vi "Target_425.vi"() -> ()   [LabVIEW 2018]
uses:
  <vilib>/Platform/TimedLoop/XDataNode/timing_clust.ctl
  <vilib>/Platform/TimedLoop/XDataNode/nitl_modes.ctl
  <vilib>/Platform/TimedLoop/XDataNode/wakeup.ctl
  <vilib>/rvi/eio/common/nirviEmuTemplateMethod_errors.vi
  <vilib>/rvi/Emulation/niFpgaSctlEmulationGetInTimedLoop.vi
  <vilib>/rvi/Emulation/niFpgaEmulationReportErrorSimple.vi
  <vilib>/rvi/Emulation/niFpgaGetClockAttributes.vi
  <vilib>/rvi/Emulation/niFpgaCriticalErrorInLSC.vi
  <vilib>/rvi/Emulation/niFpgaProcessEmulError.vi
  <vilib>/rvi/interface/RandomDataEmulation/niFpgaRandomDataHandleErrors.vi
  <vilib>/rvi/Memory/Memory_Emulation/nirvimemoryEmulation.vi
  <vilib>/rvi/Memory/Memory_Emulation/nirvimemoryFastEmulation.vi
  <vilib>/rvi/DataTransferAndStorage/Container/Common/niFpgaContainerGetUniqueNameForEmu.vi
  <vilib>/rvi/Memory/Memory_Emulation/niFpgaMemoryEmulationCacheClearOnFirstRun.vi
  <vilib>/rvi/Memory/Memory_Emulation/nirvimemoryEmulationManagerCache_MakeExclusive.vi
  <vilib>/rvi/Memory/Memory_Emulation/niFpgaMemoryEmulationValidateCache.vi
  <vilib>/rvi/Memory/Memory_Emulation/nirvimemoryEmulationManagerCache_InsertValue.vi
  <vilib>/Utility/error.llb/Clear Errors.vi
  <vilib>/rvi/Memory/Memory_Emulation/nirvimemoryEmulationManagerCache_ReleaseExclusive.vi
  <vilib>/rvi/Memory/Memory_Emulation/nirvimemoryEmulationManagerCache_GetValue.vi
  <vilib>/rvi/Emulation/niFpgaEmulationIsFPGAContextNoSignature.vi
  <vilib>/rvi/Memory/Memory_Emulation/nirvimemoryEmulationManagerCache_SetValue.vi
  <vilib>/rvi/Emulation/niFpgaSctlEmulationResourceMgr.vi
  <vilib>/eio/EIONode/EIONode.xnode
  <vilib>/Platform/TimedLoop/XDataNode/XDataNode.xnode
  <vilib>/rvi/DataTransferAndStorage/Container/XNode/niFpgaContainer.xnode
  <vilib>/rvi/interface/RandomDataEmulation/nirviRandomDataFpgaReadWriteTemplate.vi
  <vilib>/Platform/TimedLoop/XDataNode/XDNodeRunTimeDep.lvlib
  <vilib>/rvi/Memory/Memory_Emulation/niFpgaMemoryFastEmulationDramWriteAndRequestData.vi
  <vilib>/rvi/Memory/Memory_Emulation/niFpgaMemoryEmulationDramWriteAndRequestData.vi
  <instrlib>/_niInstr/Basic Elements/v1/FPGA/niInstr Basic Elements v1 FPGA.lvlib
  <vilib>/rvi/Memory/Memory_Emulation/niFpgaMemoryEmulationDramRetrieveData.vi
panel:
  in  "30":u8=30
  in  "4":u8=4
  in  "20":u8=20
  in  "3":u8=3
  in  "28":u8=28
  in  "2":u8=2
  out "XVS":bool
  out "XHS":bool
  out "TOUT0":bool
  out "TOUT1":bool
  out "TOUT2":bool
  in  "OMODE":bool
  in  "XTRIG2":bool
  in  "XTRIG1":bool
  in  "XMASTER":bool
  in  "Хватит":bool
  in  "48":bool[](array[boolean])=[FALSE, FALSE, FALSE, FALSE, FALSE, FALSE, FALSE, FALSE, FALSE, FALSE, FALSE, FALSE, FALSE, FALSE, FALSE, FALSE, FALSE, FALSE, FALSE, FALSE, FALSE, FALSE, FALSE, FALSE, FALSE, FALSE, FALSE, FALSE, FALSE, FALSE, FALSE, FALSE, FALSE, FALSE, FALSE, FALSE, FALSE, FALSE, FALSE, FALSE, FALSE, FALSE, FALSE, FALSE, FALSE, FALSE, FALSE, FALSE]
  in  "48":u8=48
  out "Записали адресов":u32
  in  "3445760":u32=3445760
  in  "Стоп":bool
  in  "4-wire":bool
  in  "W(T)/R(F)":bool
  in  "Адрес":u8
  in  "Кол-во":u16=185
  in  "185":u16=185
  in  "187":u16=187
  in  "184":u16=184
  in  "Upd_RD":bool
  in  "Upd_WR":bool
  in  "XCLR":bool
  in  "Автомат":bool
  in  "Кадр в память":bool
  in  "Кадр на ПК":bool
  in  "Нач_адр":u32
  in  "Кон_адр":u32=26920
  out "Записали FIFO":bool
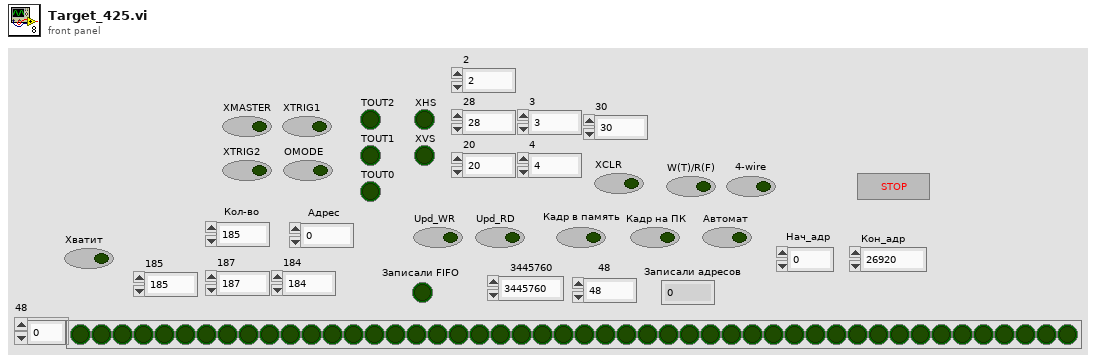
[diagram p1: front panel]
types:
  T1 = typedef "XDNodeRunTimeDep.lvlib/timing_clust.ctl" = cluster{"Expected End [f-1]":u64, "Actual End [f-1]":u64, "Finished Late? [f-1]":bool, "Expected End [i-1]":u64, "Actual End [i-1]":u64, "Finished Late? [i-1]":bool, "Expected Start [i]":u64, "Actual Start [i]":u64, "Expected Start [f]":u64, "Actual Start [f]":u64, "Source Name":string, "Structure Name":string, "Period":i64, "Deadline":i64, "Offset":i64, "Start":i64, "Priority":i32, "Timeout":i32, "Mode":T2, "Wakeup Reason":T3, "Error":errorcluster, "Source Type":string, "Secondary Source Type":string, "Global End Time":u64, "Global Start Time":u64, "Frame Duration":u64, "Iteration Duration":u64, "Assigned CPU":i32, "I/O Scan Engine Mode":u32}
  T2 = typedef "XDNodeRunTimeDep.lvlib/nitl_modes.ctl" = enum32{"No Change", "Process missed periods, maintain original phase", "Discard missed periods, maintain original phase", "Process missed periods, ignore original phase", "Discard missed periods, ignore original phase"}
  T3 = typedef "XDNodeRunTimeDep.lvlib/wakeup.ctl" = enum32{"Normal", "Aborted", "Asynchronous wakeup", "Timing source error", "Timed loop error", "Timeout"}
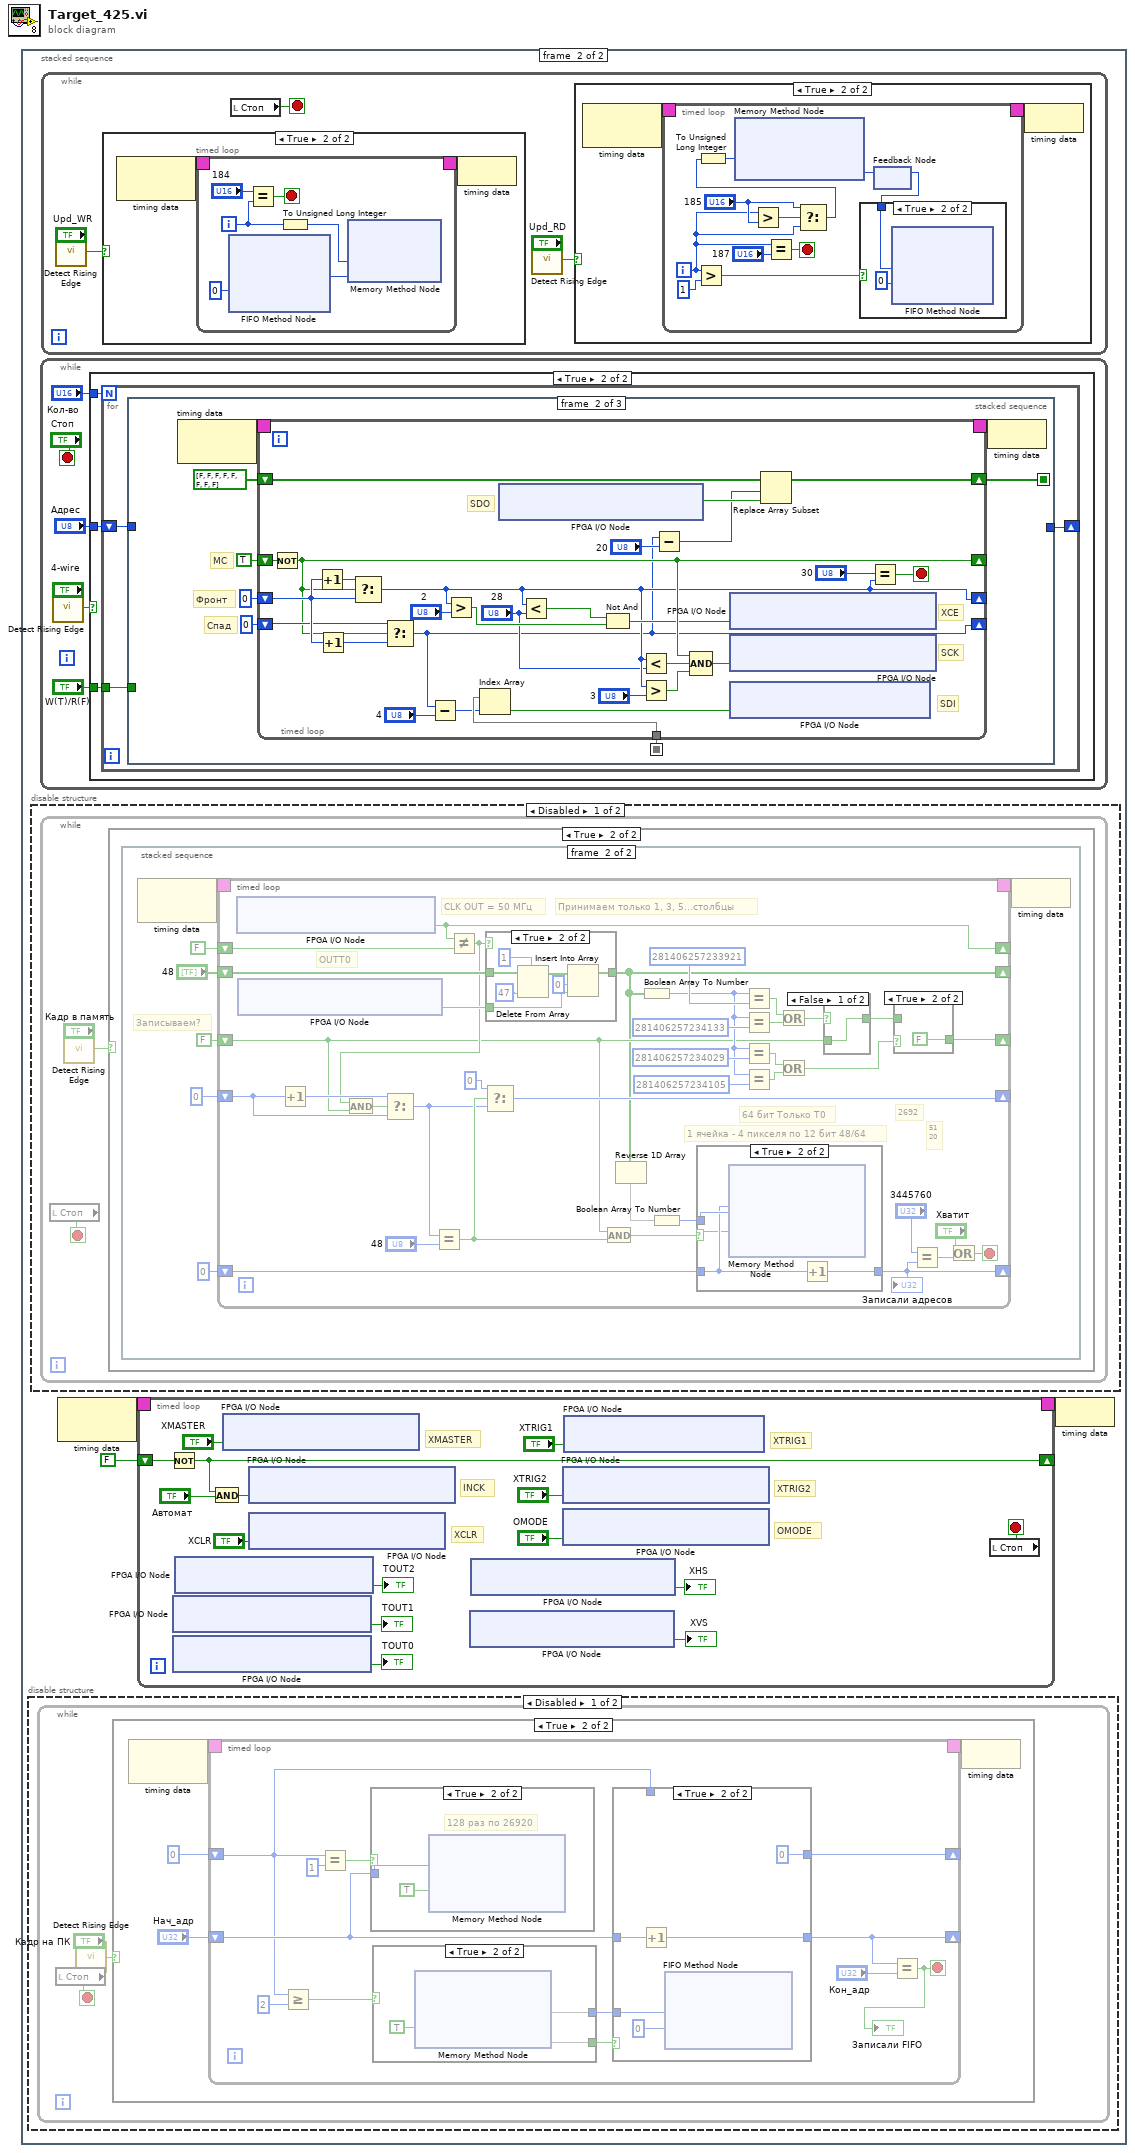
[diagram p0: block diagram]
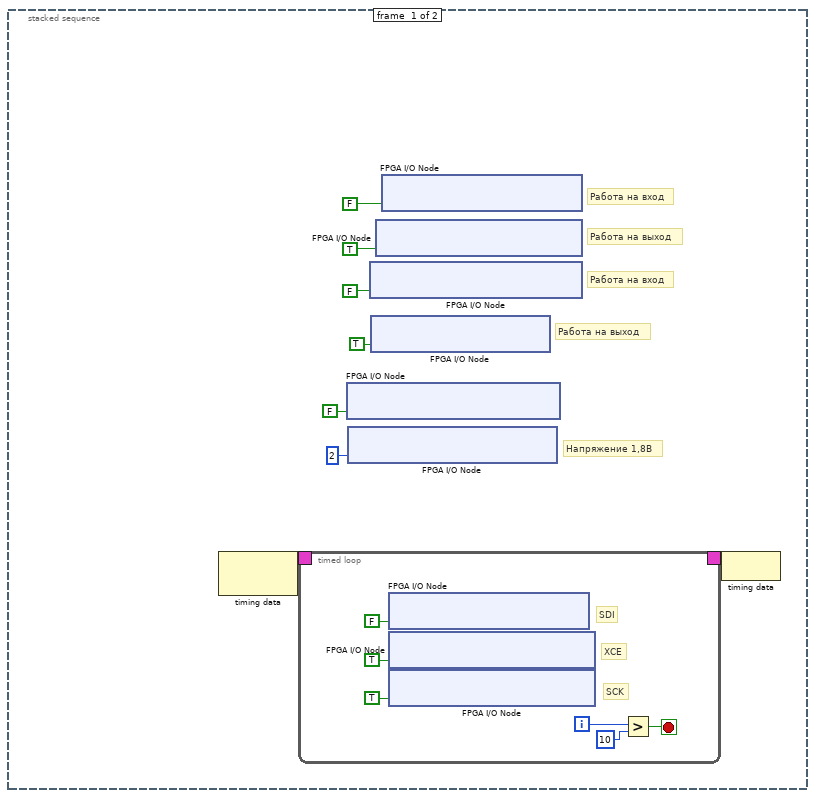
[diagram p2: hidden frame]
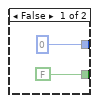
[diagram p4: hidden frame]
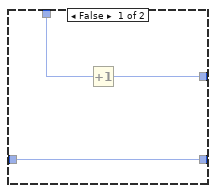
[diagram p6: hidden frame]
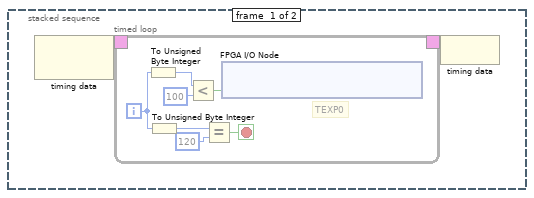
[diagram p9: hidden frame]
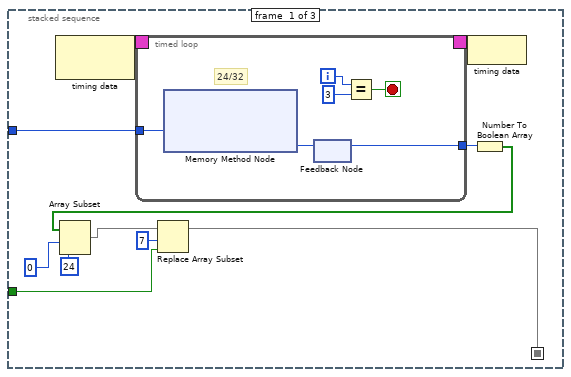
[diagram p16: hidden frame]
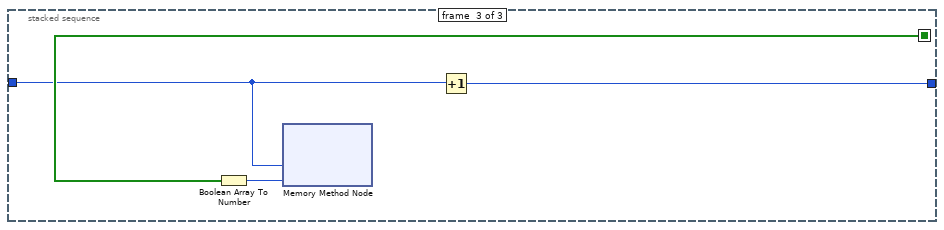
[diagram p17: hidden frame]
diagram:
  n1 = stacked-sequence {
    frame #0 {
      # "Напряжение 1,8В"
      # "Работа на выход"
      # "Работа на вход"
      # "Работа на выход"
      # "Работа на вход"
      n2 = node-c288() -> (w2:T1)  [unwired: 1 in]
      n3 = timed-loop {
        timing: w2 -> [_]
        timing-out: [_] -> w1
        i -> [w11]
        stop <- w9 stop-if-true
        # "SCK"
        # "XCE"
        # "SDI"
        n4 = xnode "FPGA I/O Node"("IO Module\\DDCA_DIO9_Write"=FALSE ("IO Module\\DDCA_DIO9_Write")) -> ()  [unwired: 1 in, 1 out]
        n5 = xnode "FPGA I/O Node"("IO Module\\DDCA_DIO13_Write"=TRUE ("IO Module\\DDCA_DIO13_Write")) -> ()  [unwired: 1 in, 1 out]
        n6 = xnode "FPGA I/O Node"("IO Module\\DDCA_DIO15_Write"=TRUE ("IO Module\\DDCA_DIO15_Write")) -> ()  [unwired: 1 in, 1 out]
        n7 = Greater?(x=w11, y=u8 10) -> (0:w9:bool)
      }
      n8 = xnode "FPGA I/O Node"("IO Module\\DDCA_Supply_Select"=FALSE ("IO Module\\DDCA_Supply_Select")) -> ()  [unwired: 1 in, 1 out]
      n9 = xnode "FPGA I/O Node"("IO Module\\Local_Supply_Select"=u8 2 ("IO Module\\Local_Supply_Select")) -> ()  [unwired: 1 in, 1 out]
      n10 = xnode "FPGA I/O Node"("IO Module\\DDCA_DIO16-23_WE"=FALSE ("IO Module\\DDCA_DIO16-23_WE")) -> ()  [unwired: 1 in, 1 out]
      n11 = xnode "FPGA I/O Node"("IO Module\\DDCA_PFI_WE"=TRUE ("IO Module\\DDCA_DIO16-23_WE")) -> ()  [unwired: 1 in, 1 out]
      n12 = xnode "FPGA I/O Node"("IO Module\\DDCA_DIO8-15_WE"=TRUE ("IO Module\\DDCA_DIO8-15_WE")) -> ()  [unwired: 1 in, 1 out]
      n13 = xnode "FPGA I/O Node"("IO Module\\DDCA_DIO0-7_WE"=FALSE ("IO Module\\DDCA_DIO0-7_WE")) -> ()  [unwired: 1 in, 1 out]
      n14 = node-c288(w1) -> ()
    }
    frame #1 {
      n15 = disable-structure shown="Disabled" {
        frame Disabled {
          n16 = while {
            stop <- w24 stop-if-true
            n17 = local read "Стоп"() -> (w24:bool)
            n18 = call <instrlib>:"Detect Rising Edge.vi"("signal"="Кадр на ПК") -> ("edge detected"=w23:bool)  [unwired: 14 in]
            n19 = case shown="True" w23 {
              frame False {
              }
              frame True {
                n20 = node-c288() -> (w28:T1)  [unwired: 1 in]
                n21 = timed-loop {
                  shift-right: [w39] -> _
                  shift-left: "Нач_адр" -> [w33]
                  timing: w28 -> [_]
                  timing-out: [_] -> w27
                  shift-right: [w31] -> _
                  shift-left: u8 0 -> [w32]
                  stop <- w40 stop-if-true
                  n22 = Greater Or Equal?(x=w32, y=u8 2 ("2")) -> (x >= y?=w34:bool)
                  n23 = Equal?(x=w32, y=u8 1 ("1")) -> (x = y?=w37:bool)
                  n24 = case shown="True" w37 {
                    tunnel: w33 -> [_ w47]
                    frame False {
                    }
                    frame True {
                      # "128 раз по 26920"
                      n25 = xnode ("Memory Method Node")("Address"=w47, "Input Valid"=TRUE) -> ()  [unwired: 1 in, 2 out]
                    }
                  }
                  n26 = case shown="True" w34 {
                    tunnel: [u8 0 ("Data") w45] -> w38
                    tunnel: [FALSE ("Output Valid") w44] -> w29
                    frame False {
                    }
                    frame True {
                      n27 = xnode ("Memory Method Node")("Ready for Output"=TRUE ("Ready For Output")) -> ("Data"=w45, "Output Valid"=w44)  [unwired: 1 in, 1 out]
                    }
                  }
                  n28 = case shown="True" w29 {
                    tunnel: [w48 w55] -> w39
                    tunnel: w38 -> [_ w52]
                    tunnel: w33 -> [w48 w54]
                    tunnel: w32 -> [w50 _]
                    tunnel: [w49 u8 0] -> w31
                    frame False {
                      n29 = Increment(x=w50) -> (x+1=w49:u8)
                    }
                    frame True {
                      n30 = Increment(x=w54) -> (x+1=w55:u32)
                      n31 = xnode ("FIFO Method Node")("Element"=w52, "Timeout"=u8 0) -> ()  [unwired: 1 in, 2 out]
                    }
                  }
                  n32 = Equal?(x=w39, y="Кон_адр") -> (x = y?=w40:bool)
                  "Записали FIFO" <- w40
                }
                n33 = node-c288(w27) -> ()
              }
            }
          }
        }
        frame Enabled {
        }
      }
      n34 = disable-structure shown="Disabled" {
        frame Disabled {
          n35 = while {
            stop <- w62 stop-if-true
            n36 = local read "Стоп"() -> (w62:bool)
            n37 = call <instrlib>:"Detect Rising Edge.vi"("signal"="Кадр в память") -> ("edge detected"=w61:bool)  [unwired: 14 in]
            n38 = case shown="True" w61 {
              frame False {
              }
              frame True {
                n39 = stacked-sequence {
                  frame #0 {
                    n40 = node-c288() -> (w64:T1)  [unwired: 1 in]
                    n41 = timed-loop {
                      timing: w64 -> [_]
                      timing-out: [_] -> w63
                      i -> [w66]
                      stop <- w68 stop-if-true
                      # "TEXP0"
                      n42 = To Unsigned Byte Integer(number=w66) -> (unsigned 8bit integer=w67:u8)
                      n43 = To Unsigned Byte Integer(number=w66) -> (unsigned 8bit integer=w65:u8)
                      n44 = Less?(x=w67, y=u8 100) -> (x < y?=w69:bool)
                      n45 = Equal?(x=w65, y=u8 120) -> (x = y?=w68:bool)
                      n46 = xnode "FPGA I/O Node"("IO Module\\DDCA_DIO4_Write"=w69) -> ()  [unwired: 1 in, 1 out]
                    }
                    n47 = node-c288(w63) -> ()
                  }
                  frame #1 {
                    # "Записываем?"
                    n48 = node-c288() -> (w82:T1)  [unwired: 1 in]
                    n49 = timed-loop {
                      shift-right: [w87] -> _
                      shift-left: FALSE -> [w119]
                      shift-right: [w89] -> _
                      shift-left: "48" -> [w116]
                      timing: w82 -> [_]
                      timing-out: [_] -> w81
                      shift-right: [w117] -> _
                      shift-left: u32 0 -> [w118]
                      shift-right: [w105] -> _
                      shift-left: FALSE -> [w92]
                      shift-right: [w95] -> _
                      shift-left: u8 0 -> [w98]
                      stop <- w86 stop-if-true
                      # "5120"
                      # "2692"
                      # "Принимаем только 1, 3, 5...столбцы"
                      # "OUTT0"
                      # "CLK OUT = 50 МГц"
                      # "1 ячейка - 4 пикселя по 12 бит 48/64"
                      # "64 бит Только T0"
                      n50 = xnode "FPGA I/O Node"() -> ("IO Module\\DDCA_DIO9_Read"=w87:bool)  [unwired: 1 in, 1 out]
                      n51 = xnode "FPGA I/O Node"() -> ("IO Module\\DDCA_DIO11_Read"=w115:bool)  [unwired: 1 in, 1 out]
                      n52 = Increment(x=w98) -> (x+1=w99:u8)
                      n53 = Not Equal?(x=w87, y=w119) -> (x != y?=w93:bool)
                      n54 = And(x=w93, y=w92) -> (x .and. y?=w91:bool)
                      n55 = Select(t=w99, s=w91, f=w98) -> (s? t:f=w94:u8)
                      n56 = Equal?(x=w94, y="48") -> (x = y?=w97:bool)
                      n57 = Select(t=u8 0, s=w97, f=w94) -> (s? t:f=w95:u8)
                      n58 = case shown="True" w93 {
                        tunnel: w116 -> [w129 w132]
                        tunnel: w115 -> [_ w135]
                        tunnel: [w129 w134] -> w89
                        frame False {
                        }
                        frame True {
                          n59 = Delete From Array(array=w132, length=u8 1, index=u8 47) -> (array with subset deleted=w133:bool[])  [unwired: 1 out]
                          n60 = Insert Into Array(array=w133, index=u8 0, new element=w135) -> (w134:bool[])
                        }
                      }
                      n61 = And(x=w92, y=w97) -> (x .and. y?=w100:bool)
                      n62 = Reverse 1D Array(array=w89) -> (reversed array=w88:bool[])
                      n63 = Boolean Array To Number(Boolean array=w89) -> (number=w102:u64)
                      n64 = Boolean Array To Number(Boolean array=w88) -> (number=w90:u64)
                      n65 = case shown="True" w100 {
                        selector: w100 -> [_ w121]
                        tunnel: [w120 w124] -> w117
                        tunnel: w90 -> [_ w123]
                        tunnel: w118 -> [w120 w122]
                        frame False {
                        }
                        frame True {
                          n66 = xnode ("Memory Method Node")("Address"=w122, "Data"=w123, "Input Valid"=w121) -> ()  [unwired: 1 in, 2 out]
                          n67 = Increment(x=w122) -> (x+1=w124:u32)
                        }
                      }
                      "Записали адресов" <- w117
                      n68 = Equal?(x=w102, y=u64 281406257233921 ("SOF")) -> (x = y?=w112:bool)
                      n69 = Equal?(x=w102, y=u64 281406257234133 ("SOL")) -> (x = y?=w111:bool)
                      n70 = Equal?(x=w102, y=u64 281406257234029 ("EOL")) -> (x = y?=w109:bool)
                      n71 = Equal?(x=w102, y=u64 281406257234105 ("EOF")) -> (x = y?=w108:bool)
                      n72 = Or(x=w112, y=w111) -> (x .or. y?=w110:bool)
                      n73 = Or(x=w109, y=w108) -> (x .or. y?=w107:bool)
                      n74 = case shown="False" w110 {
                        selector: w110 -> [_ w128]
                        tunnel: [w127 w128] -> w106
                        tunnel: w92 -> [w127 _]
                        frame False {
                        }
                        frame True {
                        }
                      }
                      n75 = case shown="True" w107 {
                        tunnel: [w125 FALSE] -> w105
                        tunnel: w106 -> [w125 _]
                        frame False {
                        }
                        frame True {
                        }
                      }
                      n76 = Equal?(x="3445760", y=w117) -> (x = y?=w84:bool)
                      n77 = Or(x="Хватит", y=w84) -> (x .or. y?=w86:bool)
                    }
                    n78 = node-c288(w81) -> ()
                  }
                }
              }
            }
          }
        }
        frame Enabled {
        }
      }
      n79 = while {
        stop <- "Стоп" stop-if-true
        n80 = call <instrlib>:"Detect Rising Edge.vi"("signal"="4-wire") -> ("edge detected"=w141:bool)  [unwired: 14 in]
        n81 = case shown="True" w141 {
          tunnel: "W(T)/R(F)" -> [_ w149]
          tunnel: "Адрес" -> [_ w148]
          tunnel: "Кол-во" -> [_ w147]
          frame False {
          }
          frame True {
            n82 = for {
              N: w147 -> [_]
              tunnel: w149 -> [w150]
              shift-right: [w151] -> _
              shift-left: w148 -> [w152]
              n83 = stacked-sequence {
                seq-local: [w153 _ _] -> [_ w177 _]
                seq-local: [_ w175 _] -> [_ _ w216]
                tunnel: w152 -> [w160 _ w214]
                tunnel: [_ _ w217] -> w151
                tunnel: w150 -> [w154 _ _]
                frame #0 {
                  n84 = node-c288() -> (w163:T1)  [unwired: 1 in]
                  n85 = timed-loop {
                    timing: w163 -> [_]
                    timing-out: [_] -> w162
                    tunnel: w160 -> [w169]
                    tunnel: [w167] -> w161
                    i -> [w166]
                    stop <- w164 stop-if-true
                    # "24/32"
                    n86 = xnode ("Memory Method Node")("Address"=w169) -> ("Data"=w168:u32)  [unwired: 1 in, 1 out]
                    n87 = feedback-in #1(w168) -> ()
                    n88 = feedback #1() -> (w167:u32)  [unwired: 1 in]
                    n89 = Equal?(x=w166, y=u8 3) -> (x = y?=w164:bool)
                  }
                  n90 = node-c288(w162) -> ()
                  n91 = Number To Boolean Array(number=w161) -> (Boolean array=w159:bool[])
                  n92 = Array Subset(array=w159, index=0, length=24) -> (w156:bool[])
                  n93 = Replace Array Subset(array=w156, new element=w154, index=7) -> (w153:bool[])
                }
                frame #1 {
                  # "Фронт"
                  # "Спад"
                  # "MC"
                  n94 = node-c288() -> (w181:T1)  [unwired: 1 in]
                  n95 = timed-loop {
                    timing: w181 -> [_]
                    timing-out: [_] -> w180
                    shift-right: [w200] -> _
                    shift-left: TRUE -> [w206]
                    shift-right: [w182] -> _
                    shift-left: u8 0 -> [w202]
                    shift-right: [w185] -> _
                    shift-left: u8 0 -> [w203]
                    tunnel: w177 -> [w195]
                    shift-right: [w208] -> w175
                    shift-left: bool[] [FALSE, FALSE, FALSE, FALSE, FALSE, FALSE, FALSE, FALSE] -> [w209]
                    stop <- w191 stop-if-true
                    # "SCK"
                    # "XCE"
                    # "SDI"
                    # "SDO"
                    n96 = Not(x=w206) -> (.not. x?=w200:bool)
                    n97 = Increment(x=w203) -> (x+1=w205:u8)
                    n98 = Increment(x=w203) -> (x+1=w204:u8)
                    n99 = Select(t=w205, s=w200, f=w203) -> (s? t:f=w185:u8)
                    n100 = Select(t=w202, s=w200, f=w204) -> (s? t:f=w182:u8)
                    n101 = Subtract(x=w182, y="4") -> (x-y=w194:u8)
                    n102 = Greater?(x=w185, y="2") -> (0:w188:bool)
                    n103 = Index Array(array=w195, index=w194) -> (element=w193:bool)
                    n104 = xnode "FPGA I/O Node"() -> ("IO Module\\DDCA_DIO16_Read"=w207:bool)  [unwired: 1 in, 1 out]
                    n105 = Less?(x=w185, y="28") -> (x < y?=w189:bool)
                    n106 = Not And(1:w188, 2:w189) -> (0:w187:bool)
                    n107 = Less?(x=w185, y="28") -> (x < y?=w198:bool)
                    n108 = Greater?(x=w185, y="3") -> (0:w197:bool)
                    n109 = Subtract(x=w182, y="20") -> (x-y=w196:u8)
                    n110 = Compound Arithmetic op=AND(w200, w198, w197) -> (w199:bool)
                    n111 = xnode "FPGA I/O Node"("IO Module\\DDCA_DIO13_Write"=w187) -> ()  [unwired: 1 in, 1 out]
                    n112 = xnode "FPGA I/O Node"("IO Module\\DDCA_DIO15_Write"=w199) -> ()  [unwired: 1 in, 1 out]
                    n113 = xnode "FPGA I/O Node"("IO Module\\DDCA_DIO9_Write"=w193) -> ()  [unwired: 1 in, 1 out]
                    n114 = Replace Array Subset(array=w209, new element=w207, index=w196) -> (w208:bool[])
                    n115 = Equal?(x="30", y=w185) -> (x = y?=w191:bool)
                  }
                  n116 = node-c288(w180) -> ()
                }
                frame #2 {
                  n117 = Boolean Array To Number(Boolean array=w216) -> (number=w215:u8)
                  n118 = xnode ("Memory Method Node")("Address"=w214, "Data"=w215) -> ()  [unwired: 2 in, 2 out]
                  n119 = Increment(x=w214) -> (x+1=w217:u8)
                }
              }
            }
          }
        }
      }
      n120 = while {
        stop <- w222 stop-if-true
        n121 = call <instrlib>:"Detect Rising Edge.vi"("signal"="Upd_WR") -> ("edge detected"=w220:bool)  [unwired: 14 in]
        n122 = case shown="True" w220 {
          frame False {
          }
          frame True {
            n123 = node-c288() -> (w243:T1)  [unwired: 1 in]
            n124 = timed-loop {
              timing: w243 -> [_]
              timing-out: [_] -> w242
              i -> [w246]
              stop <- w244 stop-if-true
              n125 = xnode ("FIFO Method Node")("Timeout"=0) -> ("Element"=w249:u32)  [unwired: 1 in, 2 out]
              n126 = Equal?(x="184", y=w246) -> (x = y?=w244:bool)
              n127 = To Unsigned Long Integer(number=w246) -> (unsigned 32bit integer=w248:u32)
              n128 = xnode ("Memory Method Node")("Address"=w248, "Data"=w249) -> ()  [unwired: 1 in, 1 out]
            }
            n129 = node-c288(w242) -> ()
          }
        }
        n130 = local read "Стоп"() -> (w222:bool)
        n131 = call <instrlib>:"Detect Rising Edge.vi"("signal"="Upd_RD") -> ("edge detected"=w218:bool)  [unwired: 14 in]
        n132 = case shown="True" w218 {
          frame False {
          }
          frame True {
            n133 = node-c288() -> (w224:T1)  [unwired: 1 in]
            n134 = timed-loop {
              timing: w224 -> [_]
              timing-out: [_] -> w223
              i -> [w227]
              stop <- w230 stop-if-true
              n135 = Greater?(x=w227, y=u8 1) -> (0:w234:bool)
              n136 = Greater?(x=w227, y="185") -> (0:w229:bool)
              n137 = Equal?(x=w227, y="187") -> (x = y?=w230:bool)
              n138 = Select(t="185", s=w229, f=w227) -> (s? t:f=w226:i32)
              n139 = To Unsigned Long Integer(number=w226) -> (unsigned 32bit integer=w233:u32)
              n140 = xnode ("Memory Method Node")("Address"=w233) -> ("Data"=w232:u8)  [unwired: 2 in, 2 out]
              n141 = feedback #2() -> (w225:u8)  [unwired: 1 in]
              n142 = case shown="True" w234 {
                tunnel: w225 -> [_ w236]
                frame False {
                }
                frame True {
                  n143 = xnode ("FIFO Method Node")("Element"=w236, "Timeout"=u8 0) -> ()  [unwired: 1 in, 2 out]
                }
              }
              n144 = feedback-in #2(w232) -> ()
            }
            n145 = node-c288(w223) -> ()
          }
        }
      }
      n146 = node-c288() -> (w21:T1)  [unwired: 1 in]
      n147 = timed-loop {
        timing: w21 -> [_]
        timing-out: [_] -> w20
        shift-right: [w263] -> _
        shift-left: FALSE -> [w267]
        stop <- w268 stop-if-true
        # "OMODE"
        # "XTRIG2"
        # "XTRIG1"
        # "XMASTER"
        # "XCLR"
        # "INCK"
        n148 = Not(x=w267) -> (.not. x?=w263:bool)
        n149 = xnode "FPGA I/O Node"() -> ("IO Module\\DDCA_DIO3_Read"=→"TOUT1":bool)  [unwired: 1 in, 1 out]
        n150 = xnode "FPGA I/O Node"() -> ("IO Module\\DDCA_DIO5_Read"=→"TOUT0":bool)  [unwired: 1 in, 1 out]
        n151 = xnode "FPGA I/O Node"() -> ("IO Module\\DDCA_DIO1_Read"=→"TOUT2":bool)  [unwired: 1 in, 1 out]
        n152 = And(x=w263, y="Автомат") -> (x .and. y?=w264:bool)
        n153 = xnode "FPGA I/O Node"("IO Module\\DDCA_PFI3_Write"="XMASTER") -> ()  [unwired: 1 in, 1 out]
        n154 = xnode "FPGA I/O Node"("IO Module\\DDCA_DIO12_Write"=w264) -> ()  [unwired: 1 in, 1 out]
        n155 = xnode "FPGA I/O Node"("IO Module\\DDCA_PFI1_Write"="XCLR") -> ()  [unwired: 1 in, 1 out]
        n156 = xnode "FPGA I/O Node"() -> ("IO Module\\DDCA_DIO20_Read"=→"XVS":bool)  [unwired: 1 in, 1 out]
        n157 = xnode "FPGA I/O Node"() -> ("IO Module\\DDCA_DIO18_Read"=→"XHS":bool)  [unwired: 1 in, 1 out]
        n158 = xnode "FPGA I/O Node"("IO Module\\DDCA_DIO10_Write"="XTRIG2") -> ()  [unwired: 1 in, 1 out]
        n159 = xnode "FPGA I/O Node"("IO Module\\DDCA_DIO11_Write"="OMODE") -> ()  [unwired: 1 in, 1 out]
        n160 = xnode "FPGA I/O Node"("IO Module\\DDCA_DIO8_Write"="XTRIG1") -> ()  [unwired: 1 in, 1 out]
        n161 = local read "Стоп"() -> (w268:bool)
      }
      n162 = node-c288(w20) -> ()
    }
  }
